vi "CreatePublicEvents.vi"(8 "error in (no error)":errorcluster, 11 "Tool Data":refnum<class "Tool Data.lvclass">) -> (0 "error out":errorcluster, 3 "Tool Data out":refnum<class "Tool Data.lvclass">)   [LabVIEW 2019, in "Tool Data.lvclass"]
doc: "---------------------------------------------------------------\nJKI State Machine Objects™\nhttp://jki.net/state-machine-objects/\nCopyright (C) 2005-2015, JKI <info@jki.net>\nALL RIGHTS RESERVEDJKI State Machine Objects (SMO) 1.0.0.4\nJKI - JKI\nCopyright (c) 2015, JKI"
uses:
  Tool Data.lvclass
  Typedefs/PublicEvents--Tool Data.Objects Updated.ctl
  Tool Path/Tool Path.lvclass
  Tool Funnel/Tool Funnel.lvclass
  Tool Rectangle/Tool Rectangle.lvclass
  Tool Dot/Tool Dots.lvclass
  Tool Data.lvclass/Tool Data.ctl
  <vilib>/JKI/JKI SMO/SMO/SMO.lvclass
panel:
  # "For instructions on how to use the JKI State Machine Objects, examples and video tutorials, visit:\nhttp://jki.net/state-machine-objects/\n\nJKI State Machine Objects™\nhttp://jki.net/state-machine-objects/\nCopyright (C) 2005-2015, JKI <info@jki.net>\nALL RIGHTS RESERVED"
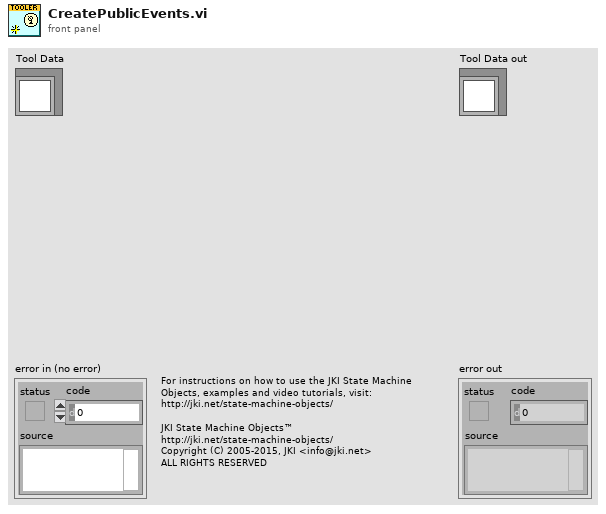
[diagram p1: front panel]
types:
  T1 = typedef "Tool Data.lvclass/PublicEvents--Tool Data.Objects Updated.ctl" = cluster{"Paths":refnum<class "Tool Path.lvclass">[], "Funnels":refnum<class "Tool Funnel.lvclass">[], "Rectangles":refnum<class "Tool Rectangle.lvclass">[], "Dots":refnum<class "Tool Dots.lvclass">[]}
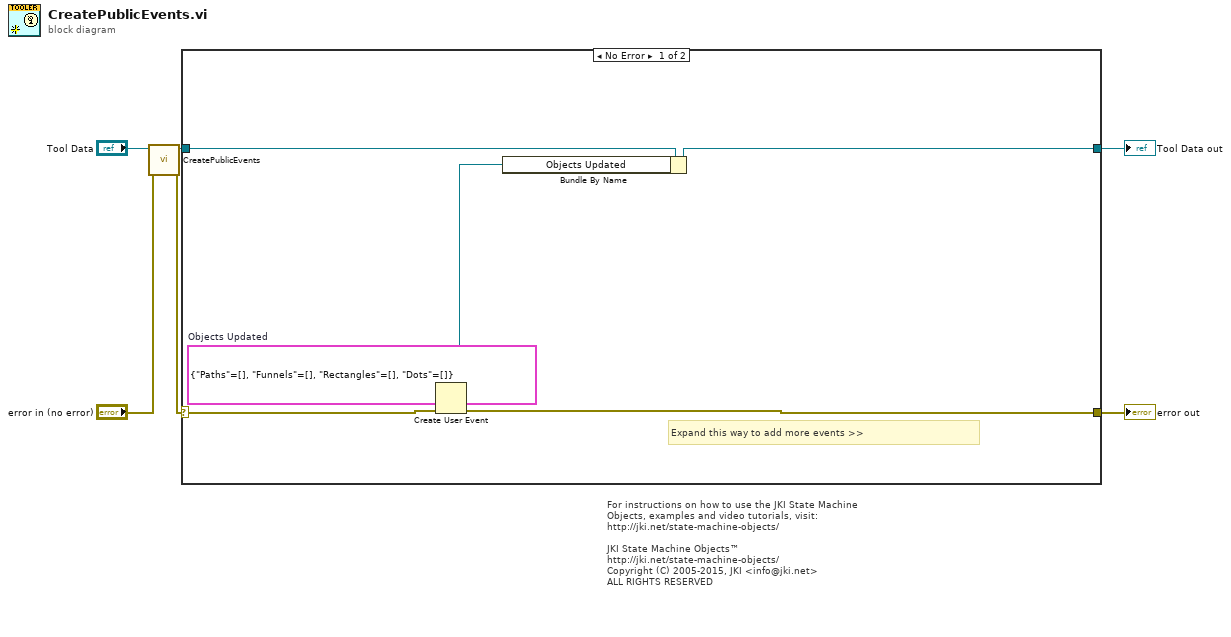
[diagram p0: block diagram]
diagram:
  # "For instructions on how to use the JKI State Machine Objects, examples and video tutorials, visit:\nhttp://jki.net/state-machine-objects/\n\nJKI State Machine Objects™\nhttp://jki.net/state-machine-objects/\nCopyright (C) 2005-2015, JKI <info@jki.net>\nALL RIGHTS RESERVED"
  n1 = call-parent "CreatePublicEvents.vi"("error in (no error)"="error in (no error)", "SMO"="Tool Data") -> ("error out"=w1:errorcluster, "SMO out"=w3:refnum<class "Tool Data.lvclass">)  [unwired: 8 in]
  n2 = case shown="No Error" w1 {
    selector: w1 -> [w11 w14]
    tunnel: [w9 w14] -> w5
    tunnel: [w10 w13] -> w6
    tunnel: w3 -> [w12 w13]
    frame No Error {
      w8 = T1 {"Paths"=[], "Funnels"=[], "Rectangles"=[], "Dots"=[]}  # Objects Updated
      # "Expand this way to add more events >>"
      n3 = Create User Event(user event datatype=w8, error in=w11) -> (user event=w7:refnum<user-event>, error out=w9:errorcluster)
      n4 = Bundle By Name(cluster=w12, "Objects Updated"=w7) -> (w10:refnum<class "Tool Data.lvclass">)
    }
    frame Error {
    }
  }
  "error out" <- w5
  "Tool Data out" <- w6
